vi "get socket option.vi"(8 "error in":errorcluster, 9 "option":i32, 10 "level":i32, 11 "s":i32) -> (0 "error out":errorcluster, 3 "option value":string)   [LabVIEW 2013, in "lvnano.lvlib"]
doc: "NN_EXPORT int nn_getsockopt (int s, int level, int option, void *optval,\n size_t *optvallen);"
uses:
  lvnano.lvlib
  get last error code.vi
  get error string from code.vi
  <vilib>/Utility/error.llb/Error Cluster From Error Code.vi
  lvnanomsg.dll
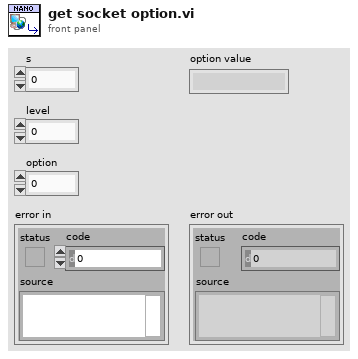
[diagram p1: front panel]
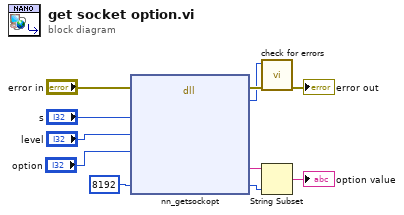
[diagram p0: block diagram]
diagram:
  n1 = dll-call lib="C:/Users/Daniel/Documents/nanomsg/lvnano/lvnanomsg.*" fn="nn_getsockopt"(error in="error in", "s"="s", "level"="level", "option"="option", "option length"=u32 8192) -> (error out=w7:errorcluster, "return type"=w5:i32, "option value"=w3:string, "option length"=w2:u32)  [unwired: 6 in, 1 out]
  n2 = call "check for errors.vi"("error in"=w7, "function return"=w5) -> ("error out"=→"error out":errorcluster)  [unwired: 9 in]
  n3 = String Subset(string=w3, length (rest)=w2) -> (substring=→"option value":string)  [unwired: 1 in]
